vi "风扇设置.vi"() -> ()   [LabVIEW 2016, in "环境动力单元.lvlib"]
uses:
  <vilib>/Utility/config.llb/NI_LVConfig.lvlib
panel:
  in  "功能开关":enum16{"关闭", "开启"}(ring)
  in  "布尔":bool
  in  "排气扇关闭温度":dbl=60.0 caption="关闭温度" format="%#_2f ℃"
  in  "排气扇开启温度":dbl=60.0 caption="开启温度" format="%#.2f ℃"
  # "参数设置"
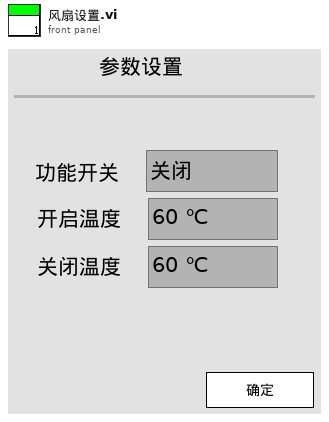
[diagram p1: front panel]
types:
  T1 = cluster{"功能开关":enum16{"关闭", "开启"}, "排气扇开启温度":dbl, "排气扇关闭温度":dbl}
  T2 = typedef "NI_LVConfig.lvlib/Config Data RefNum.ctl" = refnum<k1>
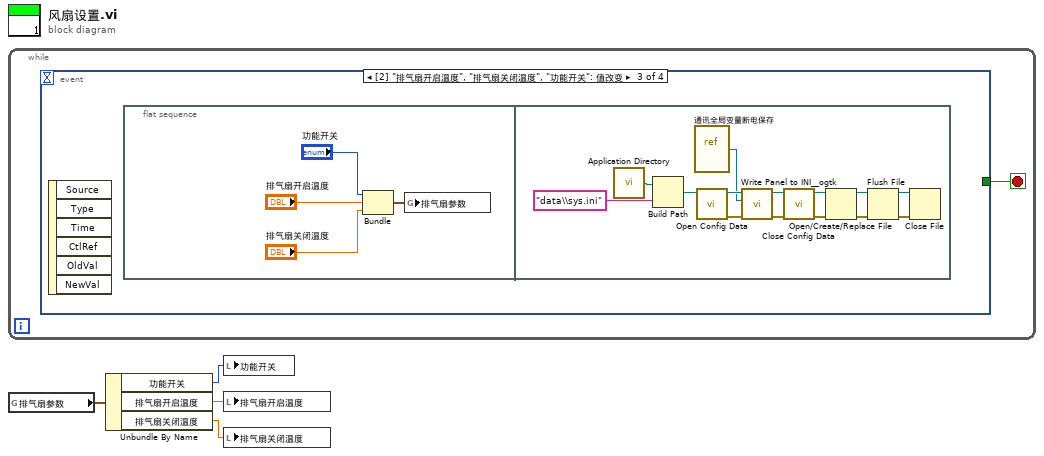
[diagram p0: block diagram]
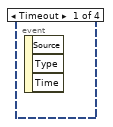
[diagram p2: hidden frame]
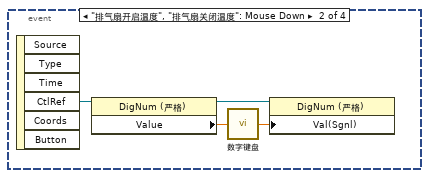
[diagram p3: hidden frame]
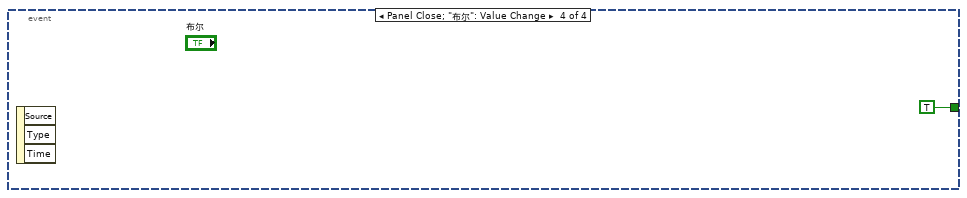
[diagram p4: hidden frame]
diagram:
  n1 = while {
    stop <- w5 stop-if-true
    n2 = event shown="[2] \"排气扇开启温度\", \"排气扇关闭温度\", \"功能开关\": 值改变" {
      selector: _ -> [_ _ _ _]
      dyn-events: _ -> [_ _ _ _]
      timeout: _ -> [_ _ _ _]
      tunnel: [_ _ _ TRUE] -> w5
      event Timeout {
        n3 = event-data() -> ()  [unwired: 1 in, 3 out]
      }
      event "排气扇开启温度", "排气扇关闭温度": Mouse Down {
        n4 = event-data() -> ("CtlRef"=w9:refnum<vi>)  [unwired: 1 in, 5 out]
        n5 = property class="DigNum (严格)"(reference=w9) -> (reference out=w6:refnum<vi>, "Value"=w8:dbl)  [unwired: 1 in, 1 out]
        n6 = call "数字键盘.vi"("OldNumber"=w8) -> ("NewNumber"=w7:dbl)
        n7 = property class="DigNum (严格)"(reference=w6, "Val(Sgnl)"=w7) -> ()  [unwired: 1 in, 2 out]
      }
      event "排气扇开启温度", "排气扇关闭温度", "功能开关": Value Change {
        n8 = event-data() -> ()  [unwired: 1 in, 6 out]
        n9 = flat-sequence {
          frame #0 {
            n10 = Bundle("功能开关"="功能开关", "排气扇开启温度"="排气扇开启温度", "排气扇关闭温度"="排气扇关闭温度") -> (w10:T1)  [unwired: 1 in]
            n11 = global write "通讯全局变量断电保存.vi" "排气扇参数"(w10) -> ()
          }
          frame #1 {
            n12 = call <vilib>:"Application Directory.vi"() -> ("Application Directory"=w27:path)
            n13 = Build Path(base path=w27, name or relative path="data\\sys.ini" ("名称或相对路径")) -> (appended path=w25:path)
            n14 = vi-ref "通讯全局变量断电保存.vi"() -> (w23:refnum<vi>)
            n15 = call <vilib>:"Open Config Data.vi"("configuration file path"=w25) -> ("error out"=w21:errorcluster, "refnum"=w24:T2)  [unwired: 8 in, 1 out]
            n16 = call <userlib>:"Write Panel to INI__ogtk.vi"("error in (no error)"=w21, "VI ref"=w23, "refnum"=w24) -> ("error out"=w20:errorcluster, "refnum out"=w22:T2)  [unwired: 7 in]
            n17 = call <vilib>:"Close Config Data.vi"("error in (no error)"=w20, "refnum"=w22) -> ("error out"=w15:errorcluster, "file path"=w14:path)  [unwired: 8 in]
            n18 = Open/Create/Replace File(file path (use dialog)=w14, error in=w15) -> (refnum out=w18:refnum<file>, error out=w19:errorcluster)  [unwired: 4 in, 1 out]
            n19 = Flush File(refnum=w18, error in=w19) -> (refnum out=w17:refnum<file>, error out=w16:errorcluster)
            n20 = Close File(refnum=w17, error in=w16) -> ()  [unwired: 2 out]
          }
        }
      }
      event Panel Close; "布尔": Value Change {
        n21 = event-data() -> ()  [unwired: 1 in, 3 out]
      }
    }
  }
  n22 = global read "通讯全局变量断电保存.vi" "排气扇参数"() -> (w4:T1)
  n23 = Unbundle By Name(w4) -> ("功能开关"=w3:enum16{"关闭", "开启"}, "排气扇开启温度"=w2:dbl, "排气扇关闭温度"=w1:dbl)
  n24 = local write "功能开关"(w3) -> ()
  n25 = local write "排气扇开启温度"(w2) -> ()
  n26 = local write "排气扇关闭温度"(w1) -> ()
